vi "SRV_Shutdown Motor Buttons.vi"(1 "button refs":refnum<vi>[](array[refnum]), 5 "false refs":refnum<vi>[](array[refnum]), 7 "true refs":refnum<vi>[](array[refnum]), 11 "error in (no error)":errorcluster) -> (15 "error out":errorcluster)   [LabVIEW 2009]
doc: "Author: Mike Schultz (LogicPD, Inc)"
uses:
  Motors Config/SRV_Motor Control Button Icons_FALSE.ctl
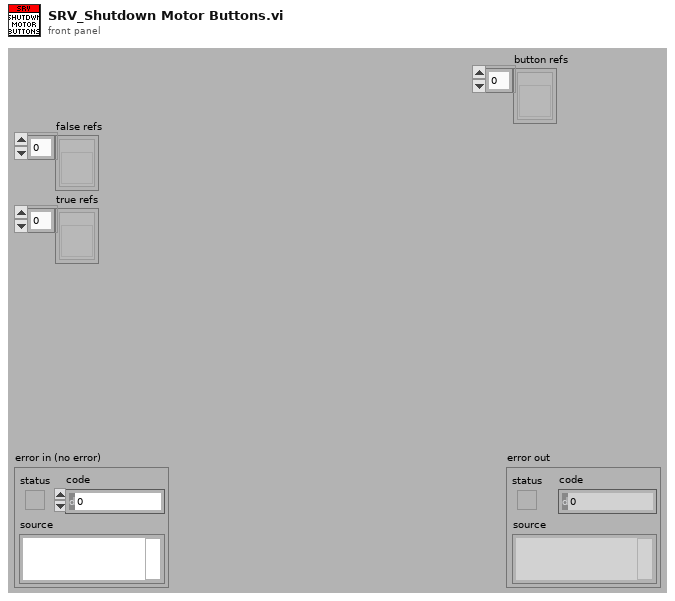
[diagram p1: front panel]
types:
  T1 = typedef "SRV_Motor Control Button Icons_FALSE.ctl" = u16
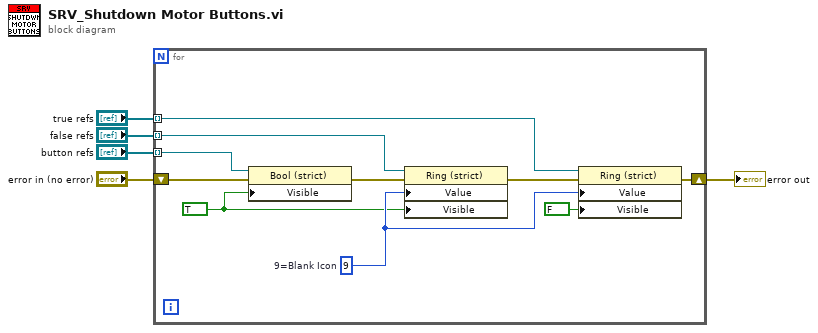
[diagram p0: block diagram]
diagram:
  n1 = for {
    tunnel: "false refs" -> [w15] mode=indexing
    shift-right: [w13] -> w3
    shift-left: "error in (no error)" -> [w10]
    tunnel: "true refs" -> [w14] mode=indexing
    tunnel: "button refs" -> [w8] mode=indexing
    w6 = TRUE ("Any Active?")
    w7 = T1 9  # 9=Blank Icon
    n2 = property class="Bool (strict)"(reference=w8, error in=w10, "Visible"=w6) -> (error out=w9:errorcluster)  [unwired: 1 out]
    n3 = property class="Ring (strict)"(reference=w15, error in=w9, "Value"=w7, "Visible"=w6) -> (error out=w11:errorcluster)  [unwired: 1 out]
    n4 = property class="Ring (strict)"(reference=w14, error in=w11, "Value"=w7, "Visible"=FALSE) -> (error out=w13:errorcluster)  [unwired: 1 out]
  }
  "error out" <- w3
